vi "Center Decoration.vi"(1 "Decoration?":bool, 2 "VI in":refnum<vi>, 4 "Object Name":string="Line Pokayoke") -> (7 "VI out":refnum<vi>)   [LabVIEW 2020]
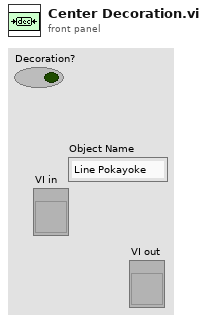
[diagram p1: front panel]
types:
  T1 = typedef "LVPointTypeDef.ctl" = cluster{"Horizontal":i16, "Vertical":i16}
  T2 = typedef "LVRectTypeDef.ctl" = cluster{"Left":i16, "Top":i16, "Right":i16, "Bottom":i16}
  T3 = typedef "LVBoundsTypeDef.ctl" = cluster{"Width":u32, "Height":u32}
  T4 = typedef "LVPositionTypeDef.ctl" = cluster{"Left":i32, "Top":i32}
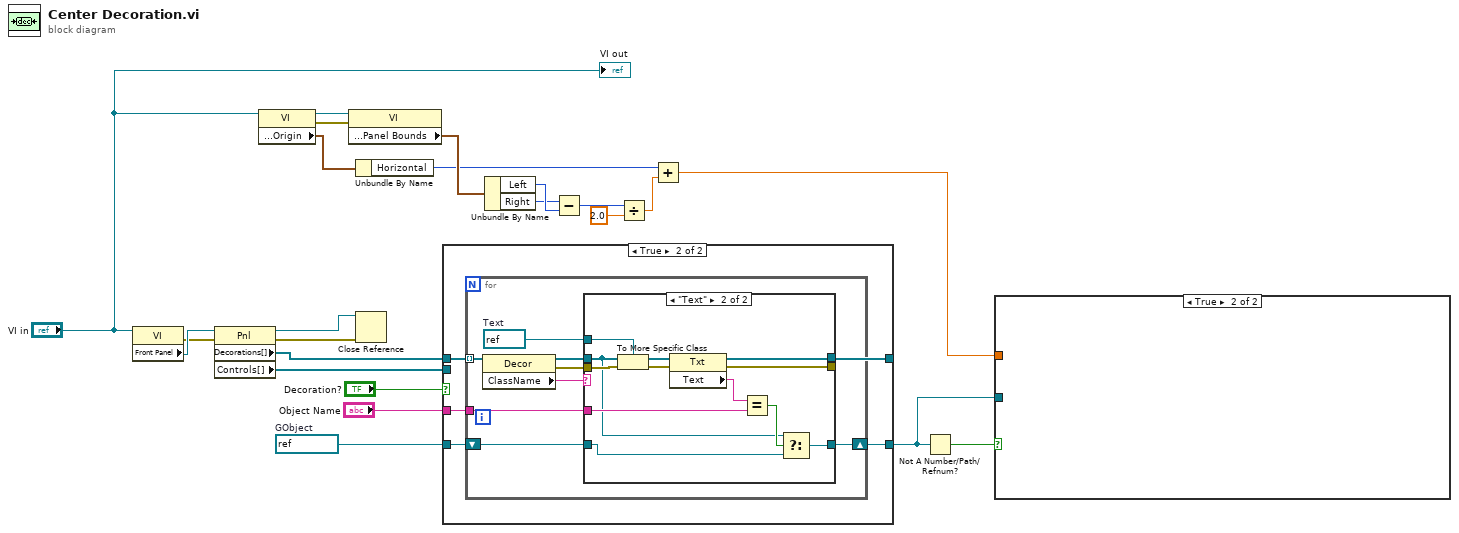
[diagram p0: block diagram]
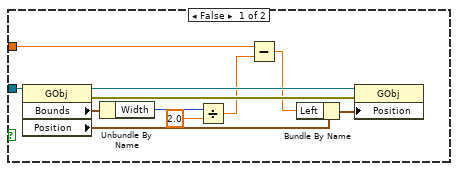
[diagram p2: hidden frame]
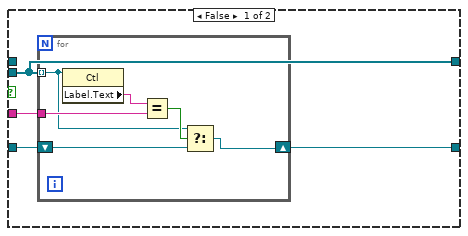
[diagram p3: hidden frame]
diagram:
  w3 = refnum<vi> refnum  # GObject
  n1 = property on="Property Node" class="VI"(reference="VI in") -> (error out=w19:errorcluster, "Front Panel"=w21:refnum<vi>)  [unwired: 1 in, 1 out]
  n2 = property on="Property Node" class="Pnl"(reference=w21, error in=w19) -> (reference out=w18:refnum<vi>, error out=w20:errorcluster, "Decorations[]"=w15:refnum<vi>[], "Controls[]"=w14:refnum<vi>[])
  n3 = property on="Property Node" class="VI"(reference="VI in") -> (reference out=w22:refnum<vi>, error out=w23:errorcluster, "Front Panel Window:Origin"=w13:T1)  [unwired: 1 in]
  n4 = property on="Property Node" class="VI"(reference=w22, error in=w23) -> ("Front Panel Window:Panel Bounds"=w7:T2)  [unwired: 2 out]
  n5 = Unbundle By Name(w13) -> ("Horizontal"=w6:i16)
  n6 = Close Reference(reference=w18, error in (no error)=w20) -> ()  [unwired: 1 out]
  n7 = case shown="True" "Decoration?" {
    tunnel: w15 -> [_ w37]
    tunnel: [w27 w37] -> _
    tunnel: w14 -> [w27 _]
    tunnel: "Object Name" -> [w26 w36]
    tunnel: [w24 w35] -> w2
    tunnel: w3 -> [w25 w34]
    frame False {
      n8 = for {
        tunnel: w27 -> [w30] mode=indexing
        tunnel: w26 -> [w32]
        shift-right: [w28] -> w24
        shift-left: w25 -> [w29]
        n9 = property class="Ctl"(reference=w30) -> ("Label.Text"=w33:string)  [unwired: 1 in, 2 out]
        n10 = Equal?(x=w33, y=w32) -> (x = y?=w31:bool)
        n11 = Select(t=w30, s=w31, f=w29) -> (s? t:f=w28:refnum<vi>)
      }
    }
    frame True {
      n12 = for {
        tunnel: w37 -> [w45] mode=indexing
        tunnel: w36 -> [w40]
        shift-right: [w39] -> w35
        shift-left: w34 -> [w38]
        w41 = refnum<vi> refnum  # Text
        n13 = property class="Decor"(reference=w45) -> (reference out=w42:refnum<vi>, error out=w43:errorcluster, "ClassName"=w44:string)  [unwired: 1 in]
        n14 = case shown="\"Text\"" w44 {
          tunnel: w43 -> [w48 w60]
          tunnel: w42 -> [w47 w51]
          tunnel: w41 -> [_ w59]
          tunnel: w40 -> [_ w55]
          tunnel: [w48 w54] -> _
          tunnel: [w47 w53] -> _
          tunnel: [w46 w49] -> w39
          tunnel: w38 -> [w46 w50]
          frame "False", Default {
          }
          frame "Text" {
            n15 = To More Specific Class(target class=w59, reference=w51, error in=w60) -> (specific class reference=w58:refnum<vi>, error out=w57:errorcluster)
            n16 = property class="Txt"(reference=w58, error in=w57) -> (reference out=w53:refnum<vi>, error out=w54:errorcluster, "Text"=w56:string)
            n17 = Equal?(x=w56, y=w55) -> (x = y?=w52:bool)
            n18 = Select(t=w51, s=w52, f=w50) -> (s? t:f=w49:refnum<vi>)
          }
        }
      }
    }
  }
  n19 = Unbundle By Name(w7) -> ("Left"=w9:i16, "Right"=w8:i16)
  n20 = Subtract(x=w8, y=w9) -> (x-y=w10:i16)
  n21 = Divide(x=w10, y=2.0) -> (x/y=w12:dbl)
  n22 = Add(x=w6, y=w12) -> (x+y=w5:dbl)
  n23 = Not A Number/Path/Refnum?(number/path/refnum=w2) -> (NaN/Path/Refnum?=w1:bool)
  n24 = case shown="True" w1 {
    tunnel: w2 -> [w71 _]
    tunnel: w5 -> [w61 _]
    frame False {
      n25 = property class="GObj"(reference=w71) -> (reference out=w68:refnum<vi>, error out=w67:errorcluster, "Bounds"=w63:T3, "Position"=w62:T4)  [unwired: 1 in]
      n26 = Unbundle By Name(w63) -> ("Width"=w70:u32)
      n27 = Divide(x=w70, y=2.0) -> (x/y=w66:dbl)
      n28 = Subtract(x=w61, y=w66) -> (x-y=w64:dbl)
      n29 = Bundle By Name(cluster=w62, "Left"=w64) -> (w65:T4)
      n30 = property class="GObj"(reference=w68, error in=w67, "Position"=w65) -> ()  [unwired: 2 out]
    }
    frame True {
    }
  }
  "VI out" <- "VI in"
